vi "Parse State Queue__jki_lib_state_machine.vi"(0 "State Queue":string, 7 "Error In (no error)":errorcluster) -> (4 "Remaining States":string, 6 "Current State":string, 8 "Arguments":string)   [LabVIEW 2020]
doc: "Parses the JKI State Machine state queue and returns the current state that will execute next with the associated arguments.\n\nFor instructions on how to use the JKI State Machine, examples and video tutorials, visit:\nhttp://jkisoft.com/state-machine/\n\n<B>Inputs:</B>\n <B>State Queue:</B> The entire state queue is wired to this input. This should come from the main JKI State Machine shift register.\n <B>Error In</B> The error cluster from the JKI State Machine is wired to this input. If an error occures and appears on this input, the current state output returns the \"Error Handler\" state.\n\n<B>Outputs:</B>\n <B>Remaining States:</B> Returns all the next states that should execute after the current state completes. These should be passed through the current state in the state machine. These can also be modified or augmented within the current state if necessary.\n <B>Current State:</B> Returns the current state that should execute next in the state machine. If an error is wired to the Error input then the current state output becomes \"Error Handler\".\n <B>Arguments:</B> Returns any argument(s) that may be used in the current state string. These arguments come after the \">>\" characters. <B>Note:</B> The arguments variable must not contain any unprintable characters like linefeed or carriage return.\n\n<B>State Syntax:</B>\nStateCategory: State >> Argument\nLine Terminator: Line feed\n <B>Example:</B>\nUI: Help >> About\n\nWhere \"UI\" is the state category\nWhere \"Help\" is the state\nWhere \"About\" is the argument\n <B>Other Examples:</B>\nApp Data: Initialize\nUI: Initialize\nHelp >> About\n\n<B>Commenting:</B>\nTo add a comment use \"//\" or \"#\" and all text to the right will be ignored\n <B>Commenting Example:</B>\nUI: Initialize // This initializes the UI\n# This whole line is a comment\n// Another comment line\n\nJKI State Machine™ 2018.0.7.45\nhttp://jki.net/state-machine/\nCopyright (C) 2005-2018, JKI <info@jki.net>\nALL RIGHTS RESERVED"
panel:
  # "For instructions on how to use the JKI State Machine, examples and video tutorials, visit:\nhttp://jki.net/state-machine/\n\nJKI State Machine™\nhttp://jki.net/state-machine/\nCopyright (C) 2005-2017, JKI <info@jki.net>\nALL RIGHTS RESERVED"
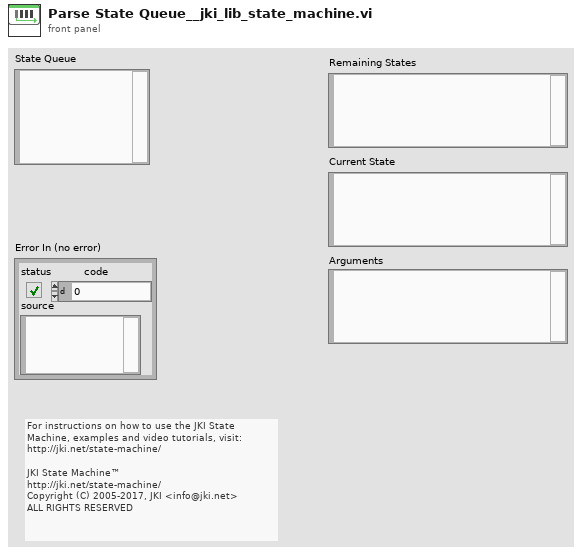
[diagram p1: front panel]
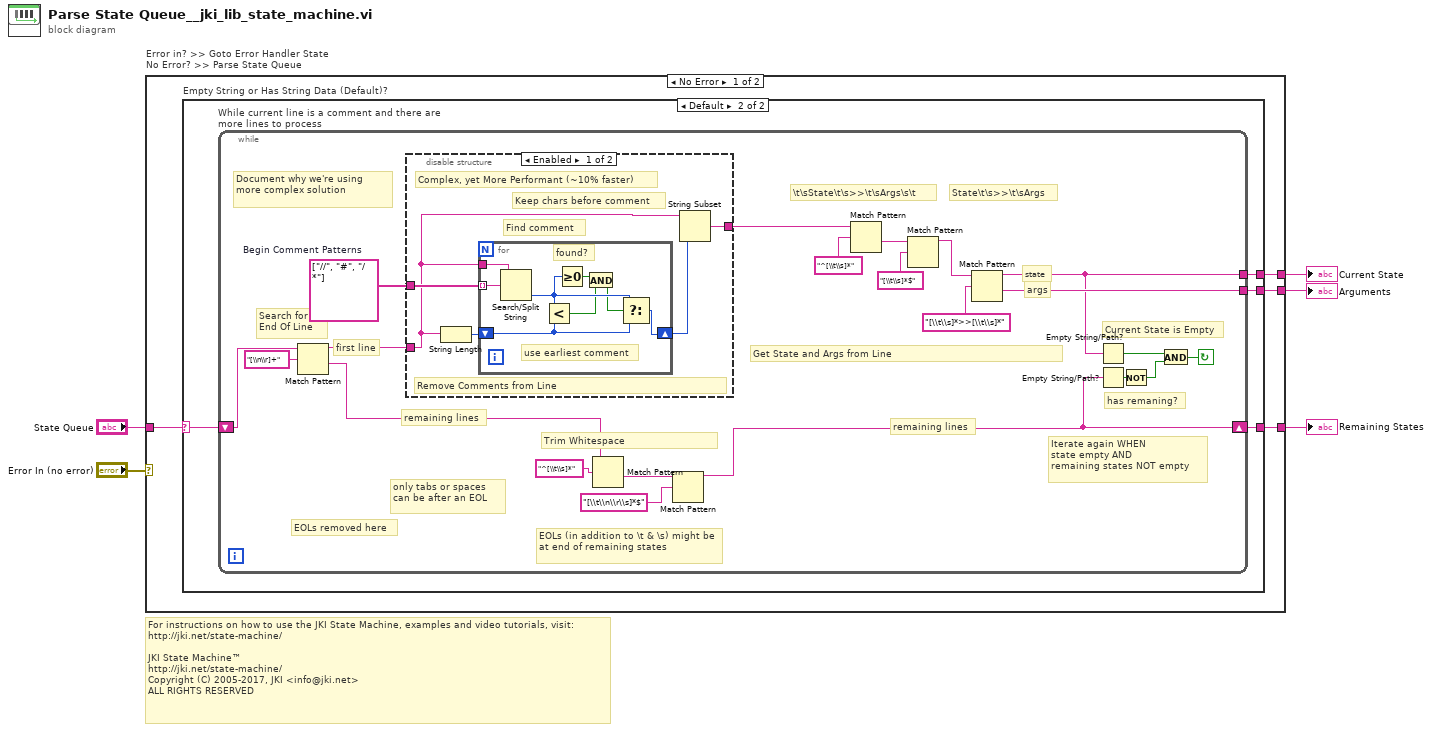
[diagram p0: block diagram]
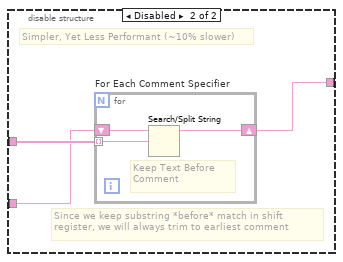
[diagram p3: hidden frame]
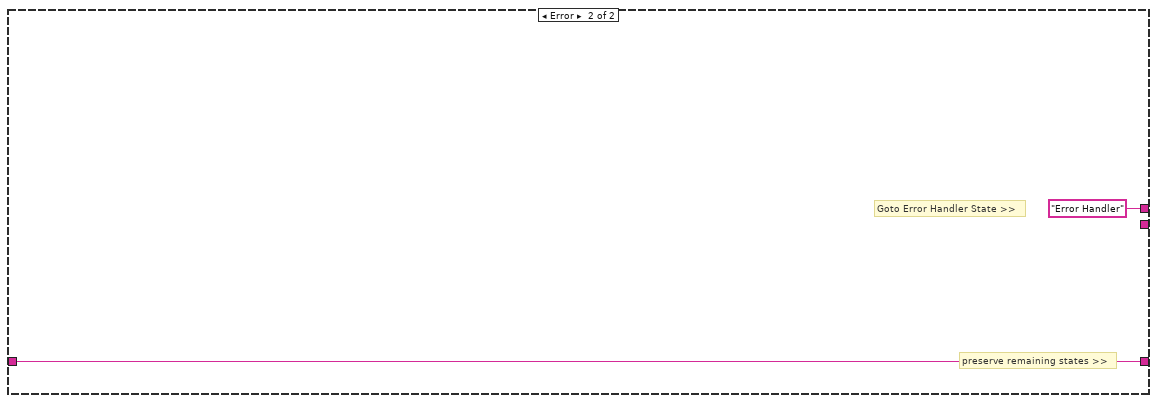
[diagram p4: hidden frame]
diagram:
  # "For instructions on how to use the JKI State Machine, examples and video tutorials, visit:\nhttp://jki.net/state-machine/\n\nJKI State Machine™\nhttp://jki.net/state-machine/\nCopyright (C) 2005-2017, JKI <info@jki.net>\nALL RIGHTS RESERVED"
  n1 = case "Error in? >> Goto Error Handler State\nNo Error? >> Parse State Queue" shown="No Error" "Error In (no error)" {
    tunnel: [w7 w55] -> w5
    tunnel: [w9 "Error Handler"] -> w3
    tunnel: [w8 _] -> w2
    tunnel: "State Queue" -> [w6 w55]
    frame No Error {
      n2 = case "Empty String or Has String Data (Default)?" shown="Default" w6 {
        selector: w6 -> [_ w10]
        tunnel: [_ w13] -> w9
        tunnel: [_ w12] -> w8
        tunnel: [_ w11] -> w7
        frame "" {
          # "Do Nothing if Empty String"
          # "<< Wiring into the Case Selector is much more performant than using \"Empty String/Path?\" primitive"
        }
        frame Default {
          n3 = while "While current line is a comment and there are more lines to process" {
            tunnel: [w33] -> w13
            tunnel: [w34] -> w12
            shift-right: [w29] -> w11
            shift-left: w10 -> [w27]
            stop <- w30 continue-if-true
            w26 = string[] ["//", "#", "/*"]  # Begin Comment Patterns
            # "Get State and Args from Line"
            # "State\\t\\s>>\\t\\sArgs"
            # "\\t\\sState\\t\\s>>\\t\\sArgs\\s\\t"
            # "remaining lines"
            # "EOLs (in addition to \\t & \\s) might be at end of remaining states"
            # "Document why we're using more complex solution"
            # "Trim Whitespace"
            # "EOLs removed here"
            # "only tabs or spaces can be after an EOL"
            # "Current State is Empty"
            # "has remaning?"
            # "remaining lines"
            # "first line"
            # "Search for End Of Line"
            # "Iterate again WHEN\nstate empty AND\nremaining states NOT empty"
            # "args"
            # "state"
            n4 = Match Pattern(string=w27, regular expression="[\\n\\r]+") -> (before substring=w24:string, after substring=w16:string)  [unwired: 1 in, 2 out]
            n5 = disable-structure shown="Enabled" {
              disable-tunnel: w26 -> [w39 w50]
              disable-tunnel: [w38 w49] -> w25
              disable-tunnel: w24 -> [w37 w48]
              frame Enabled {
                # "Remove Comments from Line"
                # "Complex, yet More Performant (~10% faster)"
                # "Keep chars before comment"
                # "Find comment"
                n6 = String Length(string=w37) -> (length=w36:i32)
                n7 = for {
                  tunnel: w39 -> [w44] mode=indexing
                  shift-right: [w46] -> w35
                  shift-left: w36 -> [w47]
                  tunnel: w37 -> [w45]
                  # "found?"
                  # "use earliest comment"
                  n8 = Search/Split String(string=w45, search string/char (-)=w44) -> (offset of match=w43:i32)  [unwired: 1 in, 2 out]
                  n9 = Less?(x=w43, y=w47) -> (x < y?=w41:bool)
                  n10 = Greater Or Equal To 0?(x=w43) -> (x >= 0?=w42:bool)
                  n11 = And(x=w42, y=w41) -> (x .and. y?=w40:bool)
                  n12 = Select(t=w43, s=w40, f=w47) -> (s? t:f=w46:i32)
                }
                n13 = String Subset(string=w37, length (rest)=w35) -> (substring=w38:string)  [unwired: 1 in]
              }
              frame Disabled {
                # "Since we keep substring *before* match in shift register, we will always trim to earliest comment"
                # "Simpler, Yet Less Performant (~10% slower)"
                n14 = for "For Each Comment Specifier" {
                  tunnel: w50 -> [w52] mode=indexing
                  shift-right: [w51] -> w49
                  shift-left: w48 -> [w53]
                  # "Keep Text Before Comment"
                  n15 = Search/Split String(string=w53, search string/char (-)=w52) -> (substring before match=w51:string)  [unwired: 1 in, 2 out]
                }
              }
            }
            n16 = Match Pattern(string=w16, regular expression="^[\\t\\s]*") -> (after substring=w15:string)  [unwired: 1 in, 3 out]
            n17 = Match Pattern(string=w15, regular expression="[\\t\\n\\r\\s]*$") -> (before substring=w29:string)  [unwired: 1 in, 3 out]
            n18 = Match Pattern(string=w25, regular expression="^[\\t\\s]*") -> (after substring=w14:string)  [unwired: 1 in, 3 out]
            n19 = Match Pattern(string=w14, regular expression="[\\t\\s]*$") -> (before substring=w18:string)  [unwired: 1 in, 3 out]
            n20 = Match Pattern(string=w18, regular expression="[\\t\\s]*>>[\\t\\s]*") -> (before substring=w33:string, after substring=w34:string)  [unwired: 1 in, 2 out]
            n21 = Empty String/Path?(string/path=w33) -> (empty?=w32:bool)
            n22 = Empty String/Path?(string/path=w29) -> (empty?=w31:bool)
            n23 = Not(x=w31) -> (.not. x?=w23:bool)
            n24 = And(x=w32, y=w23) -> (x .and. y?=w30:bool)
          }
        }
      }
    }
    frame Error {
      # "Goto Error Handler State >>"
      # "preserve remaining states >>"
    }
  }
  "Remaining States" <- w5
  "Arguments" <- w2
  "Current State" <- w3
